vi "Calc RMS V and I.vi"(11 "LAB01-1 (GRAPH)":dynamicdata(waveform)) -> (2 "RMS V":dbl, 3 "RMS I":dbl)   [LabVIEW 2017]
doc: "Calculate value of saturated waveform"
uses:
  <vilib>/measure/madcrms.llb/Basic Averaged DC-RMS for N Chan.vi
  <vilib>/measure/NI_MAPro.lvlib
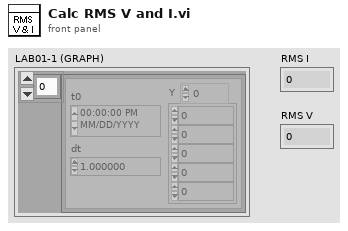
[diagram p1: front panel]
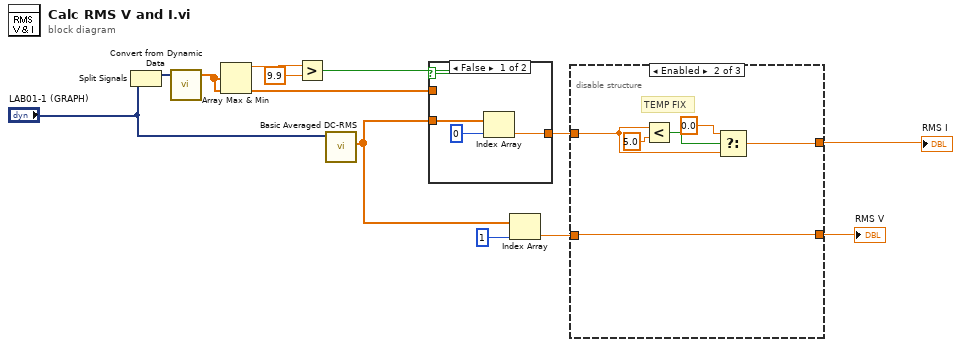
[diagram p0: block diagram]
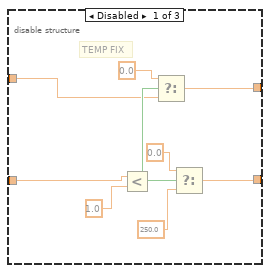
[diagram p2: hidden frame]
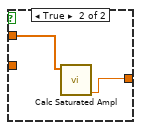
[diagram p4: hidden frame]
diagram:
  n1 = Split Signals("LAB01-1 (GRAPH)") -> (w8:dynamicdata)  [unwired: 2 in, 1 out]
  n2 = call "Convert from Dynamic Data"("Dynamic Data Type"=w8) -> ("Array"=w10:dbl[])  [unwired: 3 in]
  n3 = Array Max & Min(array=w10) -> (max value=w11:dbl)  [unwired: 3 out]
  n4 = Greater?(x=w11, y=9.9) -> (0:w9:bool)
  n5 = call-poly <vilib>:"Basic Averaged DC-RMS.vi"("signals in"="LAB01-1 (GRAPH)") -> ("RMS values"=w6:dbl[])  [unwired: 7 in, 3 out]
  n6 = case shown="False" w9 {
    tunnel: w6 -> [w15 _]
    tunnel: [w13 w16] -> w4
    tunnel: w10 -> [_ w17]
    frame False {
      n7 = Index Array(array=w15, index=0) -> (element=w13:dbl)
    }
    frame True {
      n8 = call "Calc Saturated Ampl.vi"("Waveform"=w17) -> ("RMS Amplitude"=w16:dbl)  [unwired: 5 in, 5 out]
    }
  }
  n9 = Index Array(array=w6, index=1) -> (element=w1:dbl)
  n10 = disable-structure shown="Enabled" {
    disable-tunnel: [w26 w32 w33] -> w5
    disable-tunnel: w4 -> [w20 w30 w33]
    disable-tunnel: [w19 w27 w34] -> w3
    disable-tunnel: w1 -> [w18 w27 w34]
    frame Disabled {
      # "TEMP FIX"
      n11 = Less?(x=w18, y=1.0) -> (x < y?=w21:bool)
      n12 = Select(t=0.0 ("f"), s=w21, f=w20) -> (s? t:f=w26:dbl)
      n13 = Select(t=0.0, s=w21, f=250.0) -> (s? t:f=w19:dbl)
    }
    frame Enabled {
      # "TEMP FIX"
      n14 = Less?(x=w30, y=5.0) -> (x < y?=w28:bool)
      n15 = Select(t=0.0 ("f"), s=w28, f=w30) -> (s? t:f=w32:dbl)
    }
    frame Disabled {
    }
  }
  "RMS V" <- w3
  "RMS I" <- w5
